vi "BotSpeak_AnalogOut.vi"(0 "voltage":dbl(knob) scale=0.0..5.0, 2 "Bot Settings":T1, 3 "DAC Channel":u8(slide)=3 scale=0.0..5.0) -> (1 "response":string="169.254.32.85", 4 "Bot Settings":T1)   [LabVIEW 2014]
doc: "Writes the specified \"voltage\" to the specified \"DAC Channel\"."
uses:
  <userlib>/botspeakLib/VIs/Direct/BotSpeak_Control.ctl
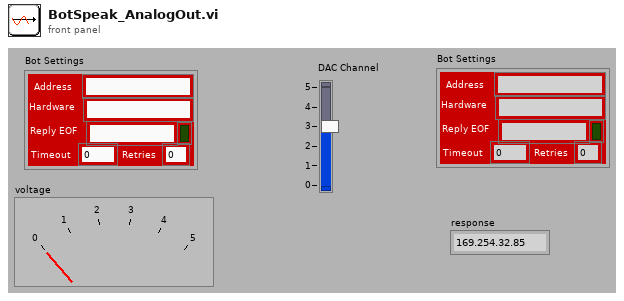
[diagram p1: front panel]
types:
  T1 = typedef "BotSpeak_Control.ctl" = cluster{"Address":string, "Reply EOF":string, "Hardware":string, "Retries":i8, "Timeout":i32, "Open?":bool}
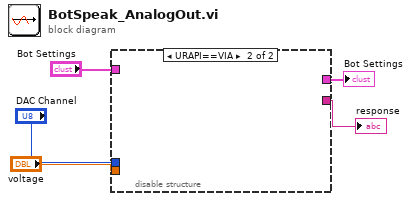
[diagram p0: block diagram]
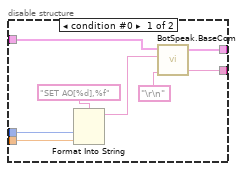
[diagram p2: hidden frame]
diagram:
  n1 = disable-structure shown="URAPI==VIA" {
    disable-tunnel: "Bot Settings" -> [w10 _]
    disable-tunnel: [w9 _] -> w4
    disable-tunnel: [w8 _] -> w3
    disable-tunnel: "DAC Channel" -> [w7 _]
    disable-tunnel: "voltage" -> [w6 _]
    frame condition #0 {
      n2 = Format Into String(format string="SET AO[%d],%f" ("command"), w7, w6) -> (resulting string=w13:string)  [unwired: 2 in, 1 out]
      n3 = call <userlib>:"BotSpeak.BaseCom.vi"("Termination"="\r\n", "command"=w13, "Bot Settings in"=w10) -> ("response"=w8:string, "Bot Settings out"=w9:T1)  [unwired: 2 in]
    }
    frame condition #1 (active) {
    }
  }
  "response" <- w3
  "Bot Settings" <- w4
